vi "Linspace.vi"(1 "NumElements":dbl=5.0, 2 "End":dbl=20.0, 3 "Start":dbl) -> (0 "Array":dbl[](array[numeric]))   [LabVIEW 2017]
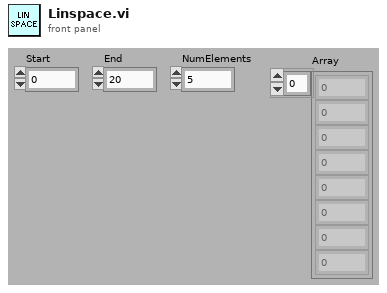
[diagram p1: front panel]
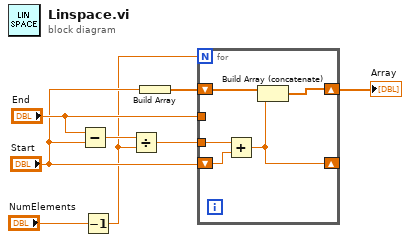
[diagram p0: block diagram]
diagram:
  n1 = Subtract(x="End", y="Start") -> (x-y=w8:dbl)
  n2 = Decrement(x="NumElements") -> (x-1=w1:dbl)
  n3 = Divide(x=w8, y=w1) -> (x/y=w7:dbl)
  n4 = Build Array("Start") -> (w5:dbl[])
  n5 = for {
    N: w1 -> [_]
    shift-right: [w10] -> w3
    shift-left: w5 -> [w13]
    tunnel: w7 -> [w12]
    tunnel: "End" -> [_]
    shift-right: [w9] -> _
    shift-left: "Start" -> [w11]
    n6 = Add(x=w12, y=w11) -> (x+y=w9:dbl)
    n7 = Build Array (concatenate)(w13, w9) -> (w10:dbl[])
  }
  "Array" <- w3
